vi "Read Key (Variant).vi"(5 "format string (%;%f)":string="%f", 7 "section":string, 8 "error in (no error)":errorcluster, 9 "type":variant, 10 "key (optional)":string, 11 "refnum":T1) -> (0 "error out":errorcluster, 1 "key-value":variant, 2 "found?":bool, 3 "refnum out":T1)   [LabVIEW 2017, in "OpenG Variant Configuration File.lvlib"]
doc: "Reads a value associated with key in a specified section of the configuration data identified by refnum. If \"key\" input is not specified, the name of the variant object is used as the key. the \"found?\" output will be TRUE for compount objects (clusters) only if all elements (recursively) are found.\n\nFor example a Boolean named \"Enable\" with a value of TRUE would correspond to the key-value pair:\n\nEnable=TRUE\n\nNote: Special characters in section and key names will be escape-coded. These include the following: \\00-\\1F (non-printable chars); \"[\", \"]\", and \"=\" (INI syntax elements); \\FE (\"þ\") and \\FF (\"ÿ\") (legacy bracket encoding); Additionally, the escape character, \"\\\", will be escaped as \"\\\\\"."
uses:
  OpenG Variant Configuration File.lvlib
  <vilib>/Utility/config.llb/Config Data RefNum.ctl
  <vilib>/Utility/Data Type/Type Definitions/Data Type.ctl
  <vilib>/Utility/config.llb/Read Key (String).vi
  <vilib>/Utility/config.llb/Read Key (Path).vi
  <vilib>/Utility/config.llb/Read Key (Boolean).vi
  <vilib>/Utility/config.llb/Read Key (Double).vi
  <vilib>/Utility/config.llb/Read Key (U32).vi
  <vilib>/Utility/config.llb/Read Key (I32).vi
  <vilib>/Utility/config.llb/NI_LVConfig.lvlib
  _openG/_reuse_openG.lvlib
  <vilib>/Utility/Data Type/NI_Data Type.lvlib
panel:
  in  "Ref for recursive call":refnum<vi>
  # "Read Key (Variant).vi\n\nReads a variant key-value from INI file.\n\nPlease visit http://www.OpenG.org to learn about the\nOpen Source LabVIEW software movement.\n\nNOTICE -- YOU MUST LEAVE THIS NOTICE IN PLACE.  PER THE TERMS OF THE LICENSE BELOW, YOU MAY SUBLICENSE THIS SOFTWARE \nIN ANY WAY THAT DOES NOT CONFLICT WITH THIS LICENSE.\n\n### BSD License (http://www.opensource.org/licenses/bsd-license.php) Begin ###\n \nCopyright (c) 2002, Jean-Pierre Drolet <drolet_jp@hotmail.com>\nCopyright (c) 2002-2006, Jim Kring <jim@jimkring.com>\n\nAll rights reserved.\n\nRedistribution and use in source and binary forms, with or without modification, are permitted provided that the following conditions are met:\n\n    * Redistributions of source code must retain the above copyright notice, this list of conditions and the following disclaimer.\n    * Redistributions in binary form must reproduce the above copyright notice, this list of conditions and the following disclaimer in the \n       documentation and/or other materials provided with the distribution.\n    * Neither the name of SciWare, James Kring, Inc., nor the names of its contributors may be used to endorse or promote products derived \n       from this software without specific prior written permission.\n\nTHIS SOFTWARE IS PROVIDED BY THE COPYRIGHT HOLDERS AND CONTRIBUTORS \"AS IS\" AND ANY EXPRESS OR IMPLIED WARRANTIES, \nINCLUDING, BUT NOT LIMITED TO, THE IMPLIED WARRANTIES OF MERCHANTABILITY AND FITNESS FOR A PARTICULAR PURPOSE ARE \nDISCLAIMED. IN NO EVENT SHALL THE COPYRIGHT OWNER OR CONTRIBUTORS BE LIABLE FOR ANY DIRECT, INDIRECT, INCIDENTAL,\n SPECIAL, EXEMPLARY, OR CONSEQUENTIAL DAMAGES (INCLUDING, BUT NOT LIMITED TO, PROCUREMENT OF SUBSTITUTE GOODS OR \nSERVICES; LOSS OF USE, DATA, OR PROFITS; OR BUSINESS INTERRUPTION) HOWEVER CAUSED AND ON ANY THEORY OF LIABILITY, \nWHETHER IN CONTRACT, STRICT LIABILITY, OR TORT (INCLUDING NEGLIGENCE OR OTHERWISE) ARISING IN ANY WAY OUT OF THE USE \nOF THIS SOFTWARE, EVEN IF ADVISED OF THE POSSIBILITY OF SUCH DAMAGE.\n\n### BSD License End ###"
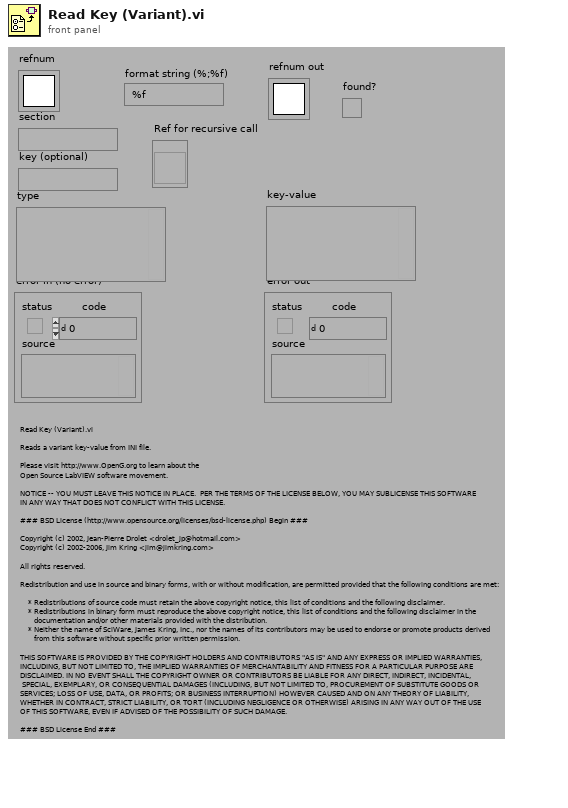
[diagram p1: front panel]
types:
  T1 = typedef "NI_LVConfig.lvlib/Config Data RefNum.ctl" = refnum<k1>
  T2 = typedef "NI_Data Type.lvlib/Data Type.ctl" = enum8{"Invalid Type", "Void", "I8", "I16", "I32", "I64", "U8", "U16", "U32", "U64", "Single Float", "Double Float", "Extended Float", "Single Complex", "Double Complex", "Extended Complex", "Enum U8", "Enum U16", "Enum U32", "Enum U64", "Single Float With Unit", "Double Float With Unit", "Extended Float With Unit", "Single Complex with Unit", "Double Complex with Unit", "Extended Complex with Unit", "Boolean", "String", "Path", "Picture", "Tag", "Array", "Cluster", "Variant", "LV Variant", "Waveform", "Timestamp", "Digital Waveform", "Digital Data", "ExpressData", "Refnum", "External Data", "VI", "Poly VI", "LabVIEW Class Instance", "Fixed Point"}
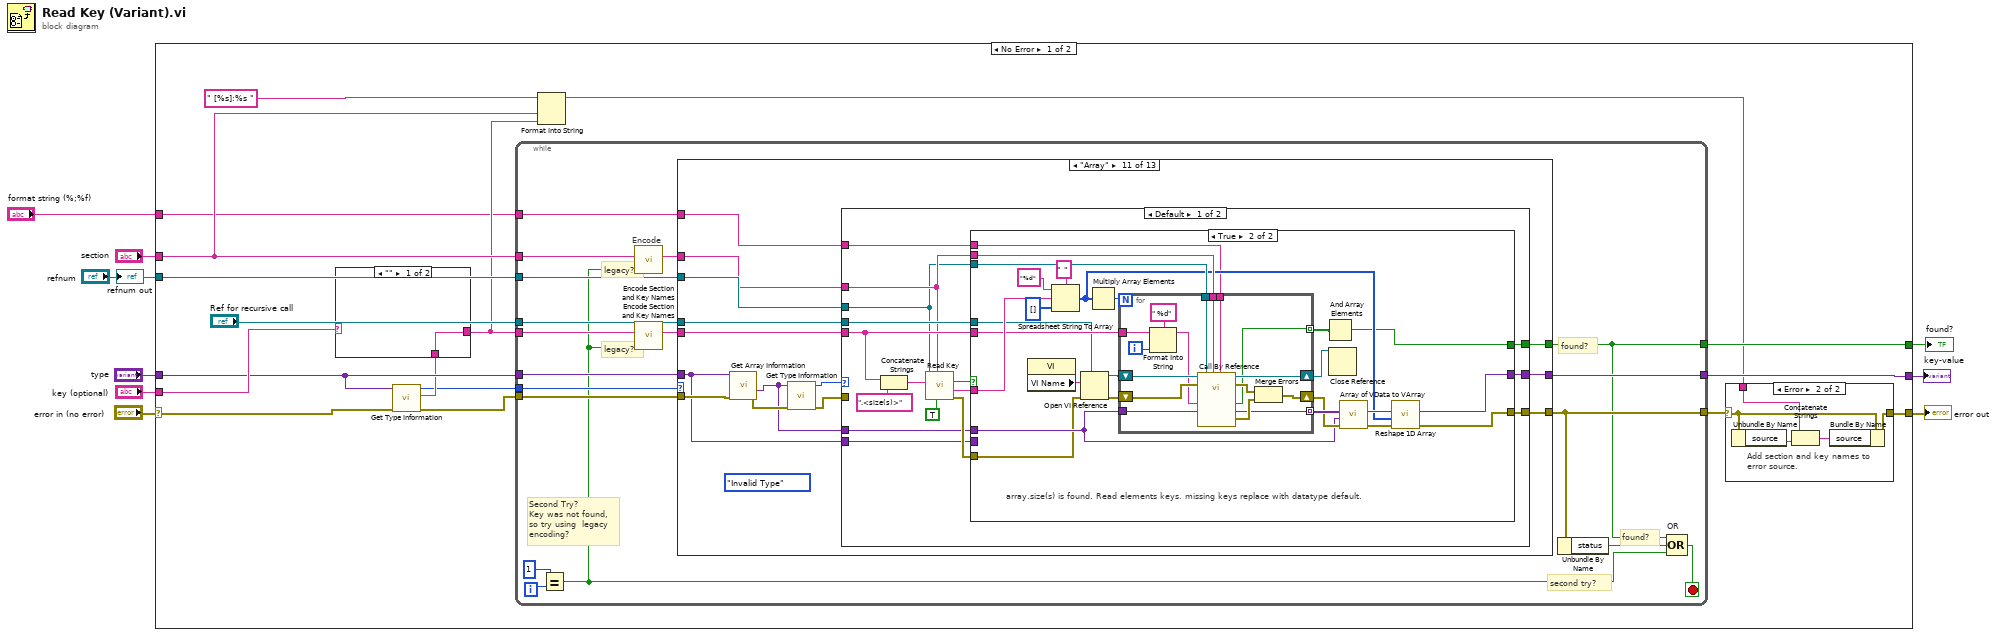
[diagram p0: block diagram]
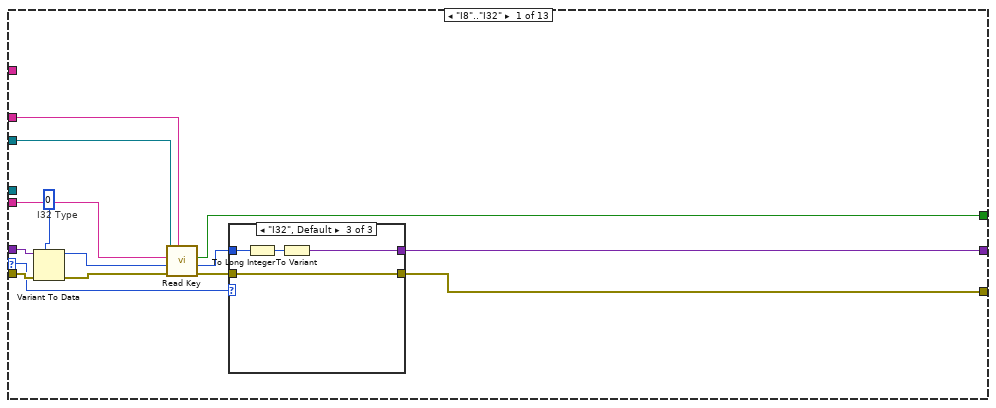
[diagram p2: hidden frame]
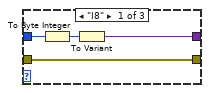
[diagram p3: hidden frame]
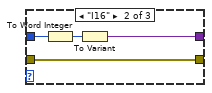
[diagram p4: hidden frame]
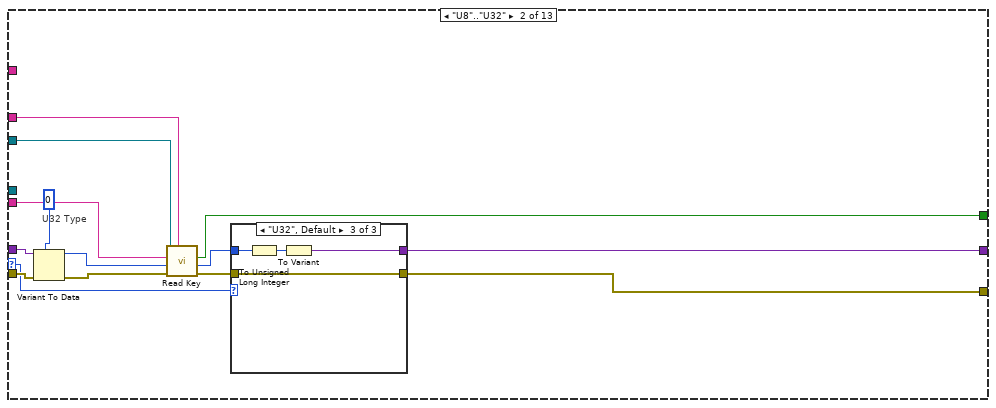
[diagram p5: hidden frame]
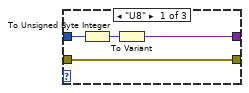
[diagram p6: hidden frame]
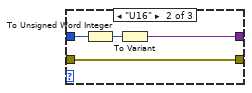
[diagram p7: hidden frame]
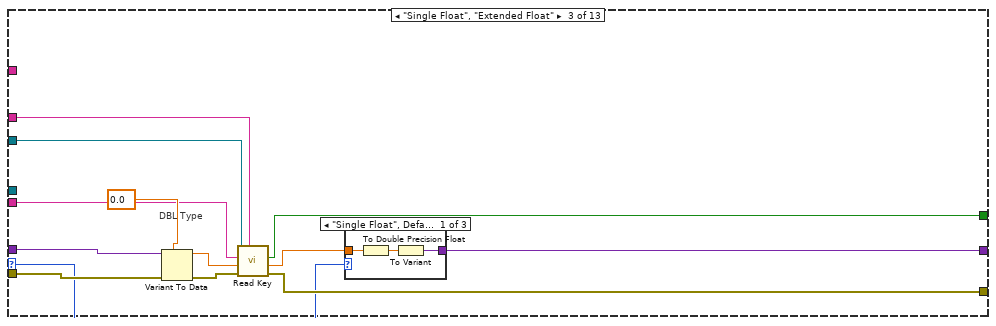
[diagram p8: hidden frame]
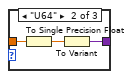
[diagram p9: hidden frame]
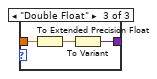
[diagram p10: hidden frame]
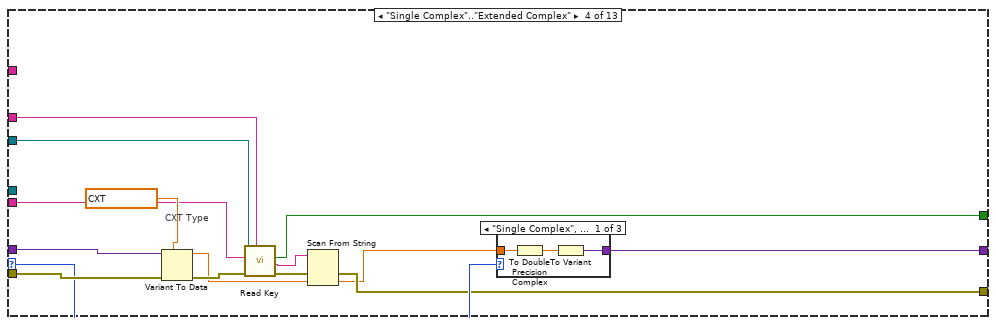
[diagram p11: hidden frame]
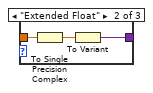
[diagram p12: hidden frame]
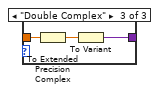
[diagram p13: hidden frame]
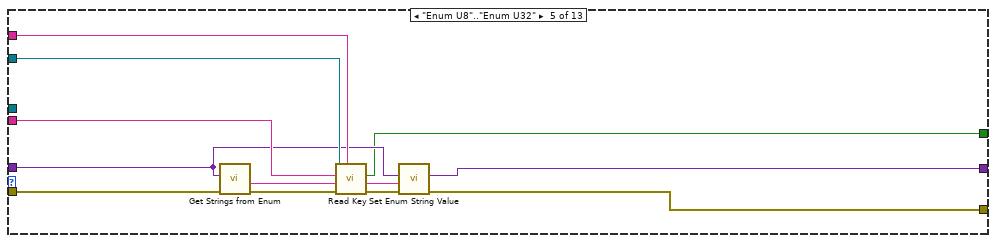
[diagram p14: hidden frame]
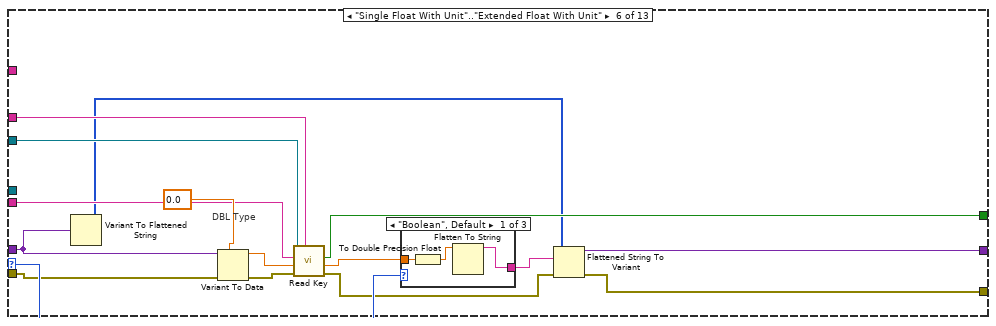
[diagram p15: hidden frame]
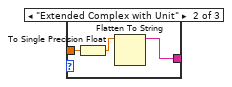
[diagram p16: hidden frame]
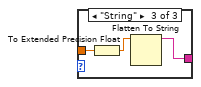
[diagram p17: hidden frame]
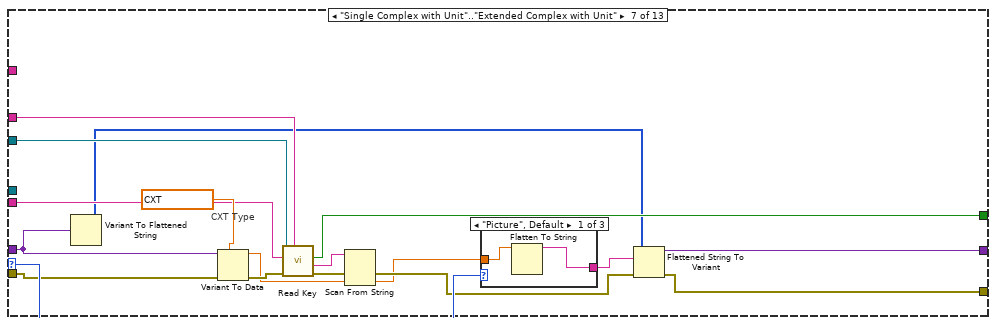
[diagram p18: hidden frame]
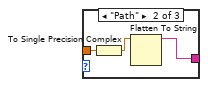
[diagram p19: hidden frame]
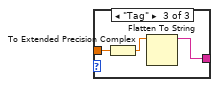
[diagram p20: hidden frame]
diagram:
  n1 = case shown="No Error" "error in (no error)" {
    selector: "error in (no error)" -> [w12 w451]
    tunnel: "refnum" -> [w26 _]
    tunnel: [w20 w451] -> w9
    tunnel: "type" -> [w13 _]
    tunnel: "key (optional)" -> [w24 _]
    tunnel: "section" -> [w17 _]
    tunnel: [w25 variant ("Variant")] -> w4
    tunnel: [w23 FALSE ("found?")] -> w2
    tunnel: "format string (%;%f)" -> [w15 _]
    frame No Error {
      n2 = call <vilib>:"Get Type Information.vi"("error in (no error)"=w12, "Variant"=w13) -> ("error out"=w14:errorcluster, "Name"=w11:string, "Type"=w10:T2)  [unwired: 5 in, 2 out]
      n3 = case shown="\"\"" w24 {
        selector: w24 -> [_ w448]
        tunnel: [w447 w448] -> w16
        tunnel: w11 -> [w447 _]
        frame "" {
        }
        frame Default {
        }
      }
      n4 = while {
        tunnel: w10 -> [w44]
        tunnel: w26 -> [w43]
        tunnel: [w42] -> w25
        tunnel: w14 -> [w41]
        tunnel: w13 -> [w40]
        tunnel: [w32] -> w23
        tunnel: "Ref for recursive call" -> [w39]
        tunnel: [w34] -> w21
        tunnel: w17 -> [w37]
        tunnel: w16 -> [w36]
        tunnel: w15 -> [w27]
        i -> [w31]
        stop <- w29 stop-if-true
        # "found?"
        # "found?"
        # "second try?"
        # "legacy?"
        # "legacy?"
        # "Second Try?\nKey was not found, so try using  legacy encoding?"
        # "Encode"
        n5 = Equal?(x=1, y=w31) -> (x = y?=w28:bool)
        n6 = call "Encode Section and Key Names.vi"("use legacy encoding scheme? (FALSE)"=w28, "string"=w37) -> ("encoded string"=w38:string)  [unwired: 9 in]
        n7 = call "Encode Section and Key Names.vi"("use legacy encoding scheme? (FALSE)"=w28, "string"=w36) -> ("encoded string"=w35:string)  [unwired: 9 in]
        n8 = case shown="\"Array\"" w44 {
          selector: w44 -> [w47 w73 w97 w124 _ w162 w191 _ _ _ _ _ _]
          tunnel: w40 -> [w57 w83 w108 w132 w145 w157 w187 w216 w228 w240 w246 w388 w437]
          tunnel: w43 -> [w56 w82 w107 w131 w154 w169 w196 w215 w227 w239 w255 w402 w440]
          tunnel: [w46 w71 w105 w122 w147 w159 w189 w213 w225 w237 w252 w391 w431] -> w34
          tunnel: w41 -> [w54 w80 w104 w129 w151 w161 w190 w212 w224 w236 w247 w390 w433]
          tunnel: w35 -> [w53 w79 w103 w128 w153 w167 w194 w211 w223 w235 w249 w400 w439]
          tunnel: w38 -> [w52 w78 w102 w127 w152 w166 w193 w210 w222 w234 w250 w401 w438]
          tunnel: [w45 w75 w99 w126 w144 w155 w185 w207 w221 w231 w253 w392 w434] -> w42
          tunnel: [w50 w74 w98 w125 w143 w163 w192 w206 w218 w230 w251 w396 w429] -> w32
          tunnel: w39 -> [_ _ _ _ _ _ _ _ _ _ w254 w395 _]
          tunnel: w27 -> [_ _ _ _ _ _ _ _ _ _ w248 w385 _]
          frame "I8".."I32" {
            # "I32 Type"
            n9 = Variant To Data(error in=w54, type=0, Variant=w57) -> (data=w51:i32, error out=w55:errorcluster)
            n10 = call-poly <vilib>:"Read Key.vi"("section"=w52, "error in (no error)"=w55, "default value"=w51, "key"=w53, "refnum"=w56) -> ("error out"=w49:errorcluster, "value"=w48:i32, "found?"=w50:bool)  [unwired: 3 in, 1 out]
            n11 = case shown="\"I32\", Default" w47 {
              tunnel: w48 -> [w62 w66 w70]
              tunnel: [w61 w65 w69] -> w45
              tunnel: w49 -> [w59 w63 w67]
              tunnel: [w59 w63 w67] -> w46
              frame "I8" {
                n12 = To Byte Integer(number=w62) -> (8bit integer=w60:i8)
                n13 = To Variant(anything=w60) -> (Variant=w61:variant)
              }
              frame "I16" {
                n14 = To Word Integer(number=w66) -> (16bit integer=w64:i16)
                n15 = To Variant(anything=w64) -> (Variant=w65:variant)
              }
              frame "I32", Default {
                n16 = To Long Integer(number=w70) -> (32bit integer=w68:i32)
                n17 = To Variant(anything=w68) -> (Variant=w69:variant)
              }
            }
          }
          frame "U8".."U32" {
            # "U32 Type"
            n18 = Variant To Data(error in=w80, type=u32 0, Variant=w83) -> (data=w77:u32, error out=w81:errorcluster)
            n19 = call-poly <vilib>:"Read Key.vi"("section"=w78, "error in (no error)"=w81, "default value"=w77, "key"=w79, "refnum"=w82) -> ("error out"=w72:errorcluster, "value"=w76:u32, "found?"=w74:bool)  [unwired: 3 in, 1 out]
            n20 = case shown="\"U32\", Default" w73 {
              tunnel: w76 -> [w88 w92 w96]
              tunnel: [w87 w91 w95] -> w75
              tunnel: w72 -> [w85 w89 w93]
              tunnel: [w85 w89 w93] -> w71
              frame "U8" {
                n21 = To Unsigned Byte Integer(number=w88) -> (unsigned 8bit integer=w86:u8)
                n22 = To Variant(anything=w86) -> (Variant=w87:variant)
              }
              frame "U16" {
                n23 = To Unsigned Word Integer(number=w92) -> (unsigned 16bit integer=w90:u16)
                n24 = To Variant(anything=w90) -> (Variant=w91:variant)
              }
              frame "U32", Default {
                n25 = To Unsigned Long Integer(number=w96) -> (unsigned 32bit integer=w94:u32)
                n26 = To Variant(anything=w94) -> (Variant=w95:variant)
              }
            }
          }
          frame "Single Float", "Extended Float" {
            # "DBL Type"
            n27 = Variant To Data(error in=w104, type=0.0, Variant=w108) -> (data=w101:dbl, error out=w106:errorcluster)
            n28 = call-poly <vilib>:"Read Key.vi"("section"=w102, "error in (no error)"=w106, "default value"=w101, "key"=w103, "refnum"=w107) -> ("error out"=w105:errorcluster, "value"=w100:dbl, "found?"=w98:bool)  [unwired: 3 in, 1 out]
            n29 = case shown="\"Single Float\", Default" w97 {
              tunnel: w100 -> [w112 w115 w118]
              tunnel: [w111 w114 w117] -> w99
              frame "Single Float", Default {
                n30 = To Double Precision Float(number=w112) -> (double precision float=w110:dbl)
                n31 = To Variant(anything=w110) -> (Variant=w111:variant)
              }
              frame "U64" {
                n32 = To Single Precision Float(number=w115) -> (single precision float=w113:sgl)
                n33 = To Variant(anything=w113) -> (Variant=w114:variant)
              }
              frame "Double Float" {
                n34 = To Extended Precision Float(1:w118) -> (0:w116:ext)
                n35 = To Variant(anything=w116) -> (Variant=w117:variant)
              }
            }
          }
          frame "Single Complex".."Extended Complex" {
            # "CXT Type"
            n36 = Variant To Data(error in=w129, type=cxt 0.0+0.0i, Variant=w132) -> (data=w120:cxt, error out=w130:errorcluster)
            n37 = call-poly <vilib>:"Read Key.vi"("section"=w127, "error in (no error)"=w130, "key"=w128, "refnum"=w131) -> ("error out"=w123:errorcluster, "value"=w121:string, "found?"=w125:bool)  [unwired: 4 in, 1 out]
            n38 = Scan From String(input string=w121, error in=w123, default 1=w120) -> (error out=w122:errorcluster, output 1=w119:cxt)  [unwired: 2 in, 2 out]
            n39 = case shown="\"Single Complex\", Default" w124 {
              tunnel: w119 -> [w136 w139 w142]
              tunnel: [w135 w138 w141] -> w126
              frame "Single Complex", Default {
                n40 = To Double Precision Complex(1:w136) -> (0:w134:cdb)
                n41 = To Variant(anything=w134) -> (Variant=w135:variant)
              }
              frame "Extended Float" {
                n42 = To Single Precision Complex(1:w139) -> (0:w137:csg)
                n43 = To Variant(anything=w137) -> (Variant=w138:variant)
              }
              frame "Double Complex" {
                n44 = To Extended Precision Complex(1:w142) -> (0:w140:cxt)
                n45 = To Variant(anything=w140) -> (Variant=w141:variant)
              }
            }
          }
          frame "Enum U8".."Enum U32" {
            n46 = call "Get Strings from Enum.vi"("error in (no error)"=w151, "Enum"=w145) -> ("error out"=w150:errorcluster, "String Value"=w149:string)  [unwired: 6 in, 2 out]
            n47 = call-poly <vilib>:"Read Key.vi"("section"=w152, "error in (no error)"=w150, "default value"=w149, "key"=w153, "refnum"=w154) -> ("error out"=w148:errorcluster, "value"=w146:string, "found?"=w143:bool)  [unwired: 3 in, 1 out]
            n48 = call "Set Enum String Value.vi"("error in (no error)"=w148, "String Value"=w146, "Default Enum Value"=w145) -> ("error out"=w147:errorcluster, "Enum"=w144:variant)  [unwired: 7 in]
          }
          frame "Single Float With Unit".."Extended Float With Unit" {
            # "DBL Type"
            n49 = Variant To Flattened String(Variant=w157) -> (1:w156:i16[])  [unwired: 1 out]
            n50 = Variant To Data(error in=w161, type=0.0, Variant=w157) -> (data=w165:dbl, error out=w168:errorcluster)
            n51 = call-poly <vilib>:"Read Key.vi"("section"=w166, "error in (no error)"=w168, "default value"=w165, "key"=w167, "refnum"=w169) -> ("error out"=w160:errorcluster, "value"=w164:dbl, "found?"=w163:bool)  [unwired: 3 in, 1 out]
            n52 = case shown="\"Boolean\", Default" w162 {
              tunnel: w164 -> [w173 w176 w179]
              tunnel: [w172 w174 w177] -> w158
              frame "Boolean", Default {
                n53 = To Double Precision Float(number=w173) -> (double precision float=w171:dbl)
                n54 = Flatten To String(anything=w171) -> (data string=w172:string)  [unwired: 3 in, 2 out]
              }
              frame "Extended Complex with Unit" {
                n55 = To Single Precision Float(number=w176) -> (single precision float=w175:sgl)
                n56 = Flatten To String(anything=w175) -> (data string=w174:string)  [unwired: 3 in, 2 out]
              }
              frame "String" {
                n57 = To Extended Precision Float(1:w179) -> (0:w178:ext)
                n58 = Flatten To String(anything=w178) -> (data string=w177:string)  [unwired: 3 in, 2 out]
              }
            }
            n59 = Flattened String To Variant(4:w160, 6:w158, 7:w156) -> (0:w159:errorcluster, 3:w155:variant)
          }
          frame "Single Complex with Unit".."Extended Complex with Unit" {
            # "CXT Type"
            n60 = Variant To Flattened String(Variant=w187) -> (1:w186:i16[])  [unwired: 1 out]
            n61 = Variant To Data(error in=w190, type=cxt 0.0+0.0i, Variant=w187) -> (data=w181:cxt, error out=w195:errorcluster)
            n62 = call-poly <vilib>:"Read Key.vi"("section"=w193, "error in (no error)"=w195, "key"=w194, "refnum"=w196) -> ("error out"=w183:errorcluster, "value"=w182:string, "found?"=w192:bool)  [unwired: 4 in, 1 out]
            n63 = Scan From String(input string=w182, error in=w183, default 1=w181) -> (error out=w184:errorcluster, output 1=w180:cxt)  [unwired: 2 in, 2 out]
            n64 = case shown="\"Picture\", Default" w191 {
              tunnel: w180 -> [w199 w202 w205]
              tunnel: [w198 w200 w203] -> w188
              frame "Picture", Default {
                n65 = Flatten To String(anything=w199) -> (data string=w198:string)  [unwired: 3 in, 2 out]
              }
              frame "Path" {
                n66 = To Single Precision Complex(1:w202) -> (0:w201:csg)
                n67 = Flatten To String(anything=w201) -> (data string=w200:string)  [unwired: 3 in, 2 out]
              }
              frame "Tag" {
                n68 = To Extended Precision Complex(1:w205) -> (0:w204:cxt)
                n69 = Flatten To String(anything=w204) -> (data string=w203:string)  [unwired: 3 in, 2 out]
              }
            }
            n70 = Flattened String To Variant(4:w184, 6:w188, 7:w186) -> (0:w189:errorcluster, 3:w185:variant)
          }
          frame "Boolean" {
            # "Boolean Type"
            n71 = Variant To Data(error in=w212, type=FALSE, Variant=w216) -> (data=w209:bool, error out=w214:errorcluster)
            n72 = call-poly <vilib>:"Read Key.vi"("section"=w210, "error in (no error)"=w214, "default value"=w209, "key"=w211, "refnum"=w215) -> ("error out"=w213:errorcluster, "value"=w208:bool, "found?"=w206:bool)  [unwired: 3 in, 1 out]
            n73 = To Variant(anything=w208) -> (Variant=w207:variant)
          }
          frame "String", "Tag" {
            # "String Type"
            n74 = Variant To Data(error in=w224, type="", Variant=w228) -> (data=w219:string, error out=w226:errorcluster)
            n75 = call-poly <vilib>:"Read Key.vi"("section"=w222, "error in (no error)"=w226, "default value"=w219, "key"=w223, "refnum"=w227) -> ("error out"=w225:errorcluster, "value"=w220:string, "found?"=w218:bool)  [unwired: 3 in, 1 out]
            n76 = To Variant(anything=w220) -> (Variant=w221:variant)
          }
          frame "Path" {
            # "Path Type"
            n77 = Variant To Data(error in=w236, type=path "", Variant=w240) -> (data=w233:path, error out=w238:errorcluster)
            n78 = call-poly <vilib>:"Read Key.vi"("section"=w234, "error in (no error)"=w238, "default value"=w233, "key"=w235, "refnum"=w239) -> ("error out"=w237:errorcluster, "value"=w232:path, "found?"=w230:bool)  [unwired: 3 in, 1 out]
            n79 = To Variant(anything=w232) -> (Variant=w231:variant)
          }
          frame "Array" {
            (unwired) Data_Type."Invalid Type" ("Type")
            n80 = call <vilib>:"Get Array Information.vi"("error in (no error)"=w247, "Variant"=w246) -> ("error out"=w245:errorcluster, "Array Element Data Type"=w242:variant)  [unwired: 6 in, 2 out]
            n81 = call <vilib>:"Get Type Information.vi"("error in (no error)"=w245, "Variant"=w242) -> ("error out"=w244:errorcluster, "Type"=w243:T2)  [unwired: 5 in, 3 out]
            n82 = case shown="Default" w243 {
              selector: w243 -> [_ w331]
              tunnel: w244 -> [_ w341]
              tunnel: w246 -> [w266 w319]
              tunnel: w250 -> [w264 w342]
              tunnel: w255 -> [w263 w343]
              tunnel: w249 -> [w267 w344]
              tunnel: w254 -> [w265 _]
              tunnel: [w261 w318] -> w253
              tunnel: [w260 errorcluster {"status"=FALSE, "code"=0, "source"=""} ("error out")] -> w252
              tunnel: [w259 w340] -> w251
              tunnel: w248 -> [w257 w316]
              tunnel: w242 -> [w256 _]
              frame Default {
                n83 = Concatenate Strings(w267, ".<size(s)>" ("Substring")) -> (w270:string)
                n84 = call-poly <vilib>:"Read Key.vi"("read raw string? (F)"=TRUE, "section"=w264, "key"=w270, "refnum"=w263) -> ("error out"=w268:errorcluster, "value"=w269:string, "found?"=w258:bool)  [unwired: 4 in, 1 out]
                n85 = case shown="True" w258 {
                  tunnel: w269 -> [_ w297]
                  tunnel: w268 -> [_ w275]
                  tunnel: w267 -> [_ w292]
                  tunnel: w266 -> [w273 _]
                  tunnel: w265 -> [_ w291]
                  tunnel: w264 -> [_ w289]
                  tunnel: w263 -> [_ w288]
                  tunnel: [w273 w281] -> w261
                  tunnel: [errorcluster {"status"=FALSE, "code"=0, "source"=""} ("error out") w280] -> w260
                  tunnel: [FALSE w278] -> w259
                  tunnel: w257 -> [_ w277]
                  tunnel: w256 -> [_ w276]
                  frame False {
                    # "array size(s) not found. Ignore element keys (if any) and return input array"
                  }
                  frame True {
                    # "array.size(s) is found. Read elements keys. missing keys replace with datatype default."
                    n86 = property class="VI"() -> ("VI Name"=w294:string)  [unwired: 2 in, 2 out]
                    n87 = Spreadsheet String To Array(delimiter (Tab)=" ", format string="%d", spreadsheet string=w297, array type (2D Dbl)=u32[] [] ("Array Constant")) -> (array=w282:u32[])
                    n88 = Open VI Reference(type specifier VI Refnum (for type only)=w291, vi path=w294, error in (no error)=w275) -> (vi reference=w290:refnum<vi>, error out=w293:errorcluster)  [unwired: 3 in]
                    n89 = Multiply Array Elements(1:w282) -> (0:w295:u32)
                    n90 = for {
                      N: w295 -> [_]
                      shift-right: [w309] -> w285
                      shift-left: w293 -> [w306]
                      shift-right: [w310] -> w287
                      shift-left: w290 -> [w308]
                      tunnel: w292 -> [w313]
                      tunnel: w276 -> [w307]
                      tunnel: w289 -> [w304]
                      tunnel: w288 -> [w303]
                      tunnel: [w302] -> w286 mode=indexing
                      tunnel: [w301] -> w279 mode=indexing
                      tunnel: w277 -> [w300]
                      i -> [w314]
                      n91 = Format Into String(format string=" %d" ("Format String"), initial string=w313, w314) -> (resulting string=w305:string)  [unwired: 1 in, 1 out]
                      n92 = call-by-ref "?"(reference=w308, error in=w306, "format string (%;%f"=w300, "section"=w304, "type"=w307, "key (optional)"=w305, "refnum"=w303) -> (reference out=w310:refnum<vi>, error out=w312:errorcluster, "error out"=w311:errorcluster, "key-value"=w302:variant, "found?"=w301:bool)  [unwired: 3 in, 1 out]
                      n93 = Merge Errors(w312, w311) -> (w309:errorcluster)
                    }
                    n94 = And Array Elements(Boolean array=w279) -> (logical AND=w278:bool)
                    n95 = Close Reference(reference=w287) -> ()  [unwired: 1 in, 1 out]
                    n96 = call "Array of VData to VArray.vi"("error in (no error)"=w285, "Element Type (when empty)"=w276, "1D Array of VData"=w286) -> ("error out"=w284:errorcluster, "VArray"=w283:variant)  [unwired: 7 in]
                    n97 = call "Reshape 1D Array.vi"("error in (no error)"=w284, "Size(s)"=w282, "1D Array"=w283) -> ("error out"=w280:errorcluster, "Reshaped VArray"=w281:variant)  [unwired: 7 in]
                  }
                }
              }
              frame "I8".."Extended Float", "Single Float With Unit".."Extended Float With Unit" {
                n98 = call-poly <vilib>:"Read Key.vi"("section"=w342, "error in (no error)"=w341, "key"=w344, "refnum"=w343) -> ("error out"=w339:errorcluster, "value"=w345:string, "found?"=w340:bool)  [unwired: 4 in, 1 out]
                n99 = Scan From String(format string="<size(s)=%[\\s0-9]> " ("regular expression"), input string=w345, error in=w339) -> (remaining string=w332:string, error out=w322:errorcluster, output 1=w337:string)  [unwired: 2 in, 1 out]
                n100 = Variant To Flattened String(Variant=w319) -> (data string=w324:string, 1:w325:i16[])
                n101 = Spreadsheet String To Array(delimiter (Tab)=" ", format string="%d", spreadsheet string=w337, array type (2D Dbl)=u32[] []) -> (array=w338:u32[])
                n102 = Type Cast(x=w338) -> (*(type *) &x=w329:string)  [unwired: 1 in]
                n103 = Spreadsheet String To Array(delimiter (Tab)=" ", format string=w316, spreadsheet string=w332, array type (2D Dbl)=dbl[] []) -> (array=w330:dbl[])
                n104 = case shown="\"U64\", \"Extended Complex with Unit\"" w331 {
                  tunnel: w330 -> [_ w352 w356 w360 w364 w368 w372 w376 w378 w382]
                  tunnel: [w347 w350 w354 w358 w362 w366 w370 w374 w380 w384] -> w327
                  tunnel: ["" w349 w353 w357 w361 w365 w369 w373 w379 w383] -> w326
                  tunnel: w329 -> [_ w349 w353 w357 w361 w365 w369 w373 w379 w383]
                  tunnel: w324 -> [w347 _ _ _ _ _ _ _ _ _]
                  frame Default {
                  }
                  frame "Void" {
                    n105 = To Byte Integer(number=w352) -> (8bit integer=w351:i8[])
                    n106 = Type Cast(x=w351) -> (*(type *) &x=w350:string)  [unwired: 1 in]
                  }
                  frame "I8" {
                    n107 = To Word Integer(number=w356) -> (16bit integer=w355:i16[])
                    n108 = Type Cast(x=w355) -> (*(type *) &x=w354:string)  [unwired: 1 in]
                  }
                  frame "I16" {
                    n109 = To Long Integer(number=w360) -> (32bit integer=w359:i32[])
                    n110 = Type Cast(x=w359) -> (*(type *) &x=w358:string)  [unwired: 1 in]
                  }
                  frame "I64" {
                    n111 = To Unsigned Byte Integer(number=w364) -> (unsigned 8bit integer=w363:u8[])
                    n112 = Type Cast(x=w363) -> (*(type *) &x=w362:string)  [unwired: 1 in]
                  }
                  frame "U8" {
                    n113 = To Unsigned Word Integer(number=w368) -> (unsigned 16bit integer=w367:u16[])
                    n114 = Type Cast(x=w367) -> (*(type *) &x=w366:string)  [unwired: 1 in]
                  }
                  frame "U16" {
                    n115 = To Unsigned Long Integer(number=w372) -> (unsigned 32bit integer=w371:u32[])
                    n116 = Type Cast(x=w371) -> (*(type *) &x=w370:string)  [unwired: 1 in]
                  }
                  frame "U64", "Extended Complex with Unit" {
                    n117 = To Single Precision Float(number=w376) -> (single precision float=w375:sgl[])
                    n118 = Type Cast(x=w375) -> (*(type *) &x=w374:string)  [unwired: 1 in]
                  }
                  frame "Single Float", "Boolean" {
                    n119 = To Double Precision Float(number=w378) -> (double precision float=w377:dbl[])
                    n120 = Type Cast(x=w377) -> (*(type *) &x=w380:string)  [unwired: 1 in]
                  }
                  frame "Double Float", "String" {
                    n121 = To Extended Precision Float(1:w382) -> (0:w381:ext[])
                    n122 = Type Cast(x=w381) -> (*(type *) &x=w384:string)  [unwired: 1 in]
                  }
                }
                n123 = Concatenate Strings(w326, w327) -> (w328:string)
                n124 = Flattened String To Variant(4:w322, 6:w328, 7:w325) -> (0:w321:errorcluster, 3:w320:variant)
                n125 = Select(t=w319, s=w321, f=w320) -> (s? t:f=w318:variant)
              }
            }
          }
          frame "Cluster" {
            # ">> Cluster Name >>"
            # "Expand cluster to its elements\nand read keys recursively."
            n126 = call "Get Data Name.vi"("error in (no error)"=w390, "Data"=w388) -> ("error out"=w389:errorcluster, "Data Name"=w386:string, "Data Dup"=w387:variant)  [unwired: 7 in]
            n127 = call "ClusterToArray.vi"("Error in"=w389, "Cluster"=w387) -> ("Error out"=w408:errorcluster, "Array"=w407:variant[])  [unwired: 8 in]
            n128 = property class="VI"() -> ("VI Name"=w406:string)  [unwired: 2 in, 2 out]
            n129 = Open VI Reference(type specifier VI Refnum (for type only)=w395, vi path=w406, error in (no error)=w408) -> (vi reference=w403:refnum<vi>, error out=w405:errorcluster)  [unwired: 3 in]
            n130 = for {
              shift-right: [w427] -> w404
              shift-left: w403 -> [w428]
              shift-right: [w412] -> w398
              shift-left: w405 -> [w423]
              tunnel: w407 -> [w421] mode=indexing
              tunnel: w401 -> [w417]
              tunnel: w402 -> [w418]
              tunnel: w400 -> [w425]
              tunnel: [w414] -> w399 mode=indexing
              tunnel: [w410] -> w397 mode=indexing
              tunnel: w385 -> [w409]
              n131 = call "Get Data Name.vi"("error in (no error)"=w423, "Data"=w421) -> ("error out"=w422:errorcluster, "Data Name"=w411:string, "Data Dup"=w420:variant)  [unwired: 7 in]
              n132 = Format Into String(format string=".%s" ("Format String"), initial string=w425, w411) -> (resulting string=w419:string)  [unwired: 1 in, 1 out]
              n133 = call-by-ref "?"(reference=w428, error in=w422, "format string (%;%f"=w409, "section"=w417, "type"=w420, "key (optional)"=w419, "refnum"=w418) -> (reference out=w427:refnum<vi>, error out=w426:errorcluster, "error out"=w416:errorcluster, "key-value"=w415:variant, "found?"=w410:bool)  [unwired: 3 in, 1 out]
              n134 = Merge Errors(w426, w416) -> (w413:errorcluster)
              n135 = call "Set Data Name.vi"("error in (no error)"=w413, "Data Name"=w411, "Data"=w415) -> ("error out"=w412:errorcluster, "Renamed Data"=w414:variant)  [unwired: 7 in]
            }
            n136 = And Array Elements(Boolean array=w397) -> (logical AND=w396:bool)
            n137 = call "ArrayToCluster.vi"("Error in"=w398, "Array"=w399) -> ("Error out"=w394:errorcluster, "Cluster"=w393:variant)  [unwired: 8 in]
            n138 = Close Reference(reference=w404) -> ()  [unwired: 1 in, 1 out]
            n139 = call "Set Data Name.vi"("error in (no error)"=w394, "Data Name"=w386, "Data"=w393) -> ("error out"=w391:errorcluster, "Renamed Data"=w392:variant)  [unwired: 7 in]
          }
          frame Default {
            n140 = Variant To Flattened String(Variant=w437) -> (data string=w436:string, 1:w430:i16[])
            n141 = call-poly <vilib>:"Read Key.vi"("section"=w438, "error in (no error)"=w433, "default value"=w436, "key"=w439, "refnum"=w440) -> ("error out"=w432:errorcluster, "value"=w435:string, "found?"=w429:bool)  [unwired: 3 in, 1 out]
            n142 = Flattened String To Variant(4:w432, 6:w435, 7:w430) -> (0:w431:errorcluster, 3:w434:variant)
          }
        }
        n143 = Unbundle By Name(w34) -> ("status"=w33:bool)
        n144 = Compound Arithmetic op=OR "OR"(w32, w33, w28) -> (w29:bool)
      }
      n145 = Format Into String(format string=" [%s]:%s " ("Format String"), w17, w16) -> (resulting string=w18:string)  [unwired: 2 in, 1 out]
      n146 = case shown="Error" w21 {
        selector: w21 -> [w441 w446]
        tunnel: [w441 w445] -> w20
        tunnel: w18 -> [_ w442]
        frame No Error {
        }
        frame Error {
          # "Add section and key names to\nerror source."
          n147 = Unbundle By Name(w446) -> ("source"=w443:string)
          n148 = Concatenate Strings(w442, w443) -> (w444:string)
          n149 = Bundle By Name(cluster=w446, "source"=w444) -> (w445:errorcluster)
        }
      }
    }
    frame Error {
    }
  }
  "error out" <- w9
  "key-value" <- w4
  "found?" <- w2
  "refnum out" <- "refnum"
